vi "Inverse Filter Demo.vi"() -> ()   [LabVIEW 2015]
uses:
  Calibration VIs/Inverse Filter VIs/InvFilt-Params.ctl
  <vilib>/sound2/lvsound2.llb/Sampling Mode.ctl
  <vilib>/sound2/lvsound2.llb/Sound Data Format.ctl
  <vilib>/sound2/lvsound2.llb/Sound Output Write (DBL Single).vi
panel:
  out "Numeric":i32
  out "Waveform Graph":dbl[](graph)
  in  "stop":bool
  in  "InvFilt Params":T1={"Min Frequency (Hz)"=1000.0, "Max Frequency (Hz)"=100000.0, "Length (points)"=301, "Sampling rate (Hz)"=100000.0, "Delay (ms)"=1.5, "Linear phase"=FALSE}
  in  "T (s)":dbl=0.5
  in  "Calibration file":path=path "U:/Shared/Hancock/Test Data/Data/RightPrimary.calib"
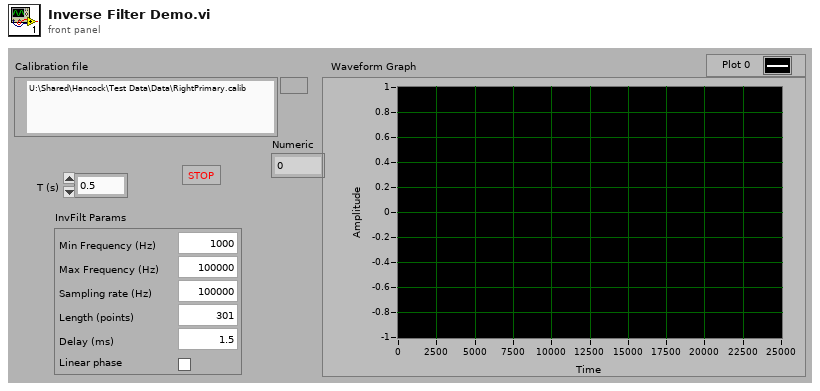
[diagram p1: front panel]
types:
  T1 = typedef "InvFilt-Params.ctl" = cluster{"Min Frequency (Hz)":dbl, "Max Frequency (Hz)":dbl, "Length (points)":i32, "Sampling rate (Hz)":dbl, "Delay (ms)":dbl, "Linear phase":bool}
  T2 = typedef "Sound Data Format.ctl" = cluster{"sample rate (S/s)":dbl, "number of channels":i32, "bits per sample":i32}
  T3 = typedef "Sampling Mode.ctl" = i32
  T4 = typedef "Sound Output Task ID.ctl" = u32
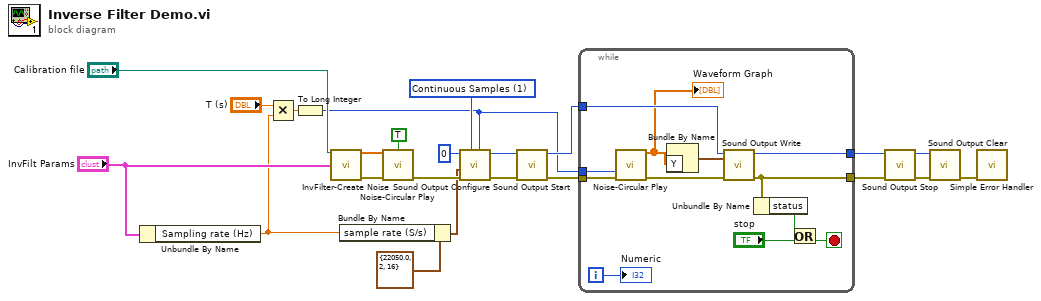
[diagram p0: block diagram]
diagram:
  w15 = T3 1 items=["Finite Samples", "Continuous Samples"] ("sample mode")
  n1 = Unbundle By Name("InvFilt Params") -> ("Sampling rate (Hz)"=w12:dbl)
  n2 = Multiply(x="T (s)", y=w12) -> (x*y=w23:dbl)
  n3 = To Long Integer(number=w23) -> (32bit integer=w2:i32)
  n4 = call "InvFilter-Create Noise.vi"("Calibration File"="Calibration file", "InvFilt Params"="InvFilt Params") -> ("InvFilter Noise"=w20:dbl[], "error out"=w19:errorcluster)  [unwired: 10 in, 2 out]
  n5 = Bundle By Name(cluster=T2 {"sample rate (S/s)"=22050.0, "number of channels"=2, "bits per sample"=16} ("sound format"), "sample rate (S/s)"=w12) -> (w11:T2)
  n6 = call "Noise-Circular Play.vi"("Noise (in)"=w20, "Init? (F)"=TRUE ("Init?"), "error in (no error)"=w19) -> ("error out"=w17:errorcluster)  [unwired: 11 in, 1 out]
  n7 = call <vilib>:"Sound Output Configure.vi"("number of samples/ch"=w2, "sample mode"=w15, "error in (no error)"=w17, "sound format"=w11, "device ID"=u32 0) -> ("error out"=w6:errorcluster, "task ID"=w5:T4)  [unwired: 5 in]
  n8 = call <vilib>:"Sound Output Start.vi"("error in (no error)"=w6, "task ID"=w5) -> ("error out"=w4:errorcluster, "task ID out"=w3:T4)  [unwired: 8 in]
  n9 = while {
    tunnel: w4 -> [w35]
    tunnel: w3 -> [w33]
    tunnel: [w26] -> w10
    tunnel: [w30] -> w9
    tunnel: w2 -> [w28]
    i -> [w24]
    stop <- w27 stop-if-true
    n10 = call "Noise-Circular Play.vi"("Npts"=w28, "error in (no error)"=w35) -> ("Noise (out)"=w29:dbl[], "error out"=w34:errorcluster)  [unwired: 12 in]
    "Waveform Graph" <- w29
    n11 = Bundle By Name("Y"=w29) -> (w32:waveform(dbl))  [unwired: 1 in]
    n12 = call-poly <vilib>:"Sound Output Write.vi"("error in (no error)"=w34, "data"=w32, "task ID"=w33) -> ("error out"=w26:errorcluster, "task ID out"=w30:T4)  [unwired: 7 in]
    n13 = Unbundle By Name(w26) -> ("status"=w25:bool)
    n14 = Or(x=w25, y="stop") -> (x .or. y?=w27:bool)
    "Numeric" <- w24
  }
  n15 = call <vilib>:"Sound Output Stop.vi"("error in (no error)"=w10, "task ID"=w9) -> ("error out"=w8:errorcluster, "task ID out"=w7:T4)  [unwired: 8 in]
  n16 = call <vilib>:"Sound Output Clear.vi"("error in (no error)"=w8, "task ID"=w7) -> ("error out"=w1:errorcluster)  [unwired: 9 in]
  n17 = call <vilib>:"Simple Error Handler.vi"("error in (no error)"=w1) -> ()  [unwired: 4 in, 5 out]
